vi "ziGetCurrentCalc.vi"   [LabVIEW 2015, in "Zurich Instruments LabOne.lvlib"]
uses:
  Zurich Instruments LabOne.lvlib
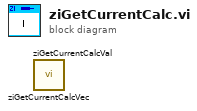
[diagram p0: block diagram]
diagram:
  n1 = call "ziGetCurrentCalcVec.vi"() -> ()  [unwired: 11 in, 1 out]
  n2 = call "ziGetCurrentCalcVal.vi"() -> ()  [unwired: 11 in, 1 out]
